vi "4.2.vi"() -> ()   [LabVIEW 2016]
panel:
  out "波形图":dbl[][](graph)
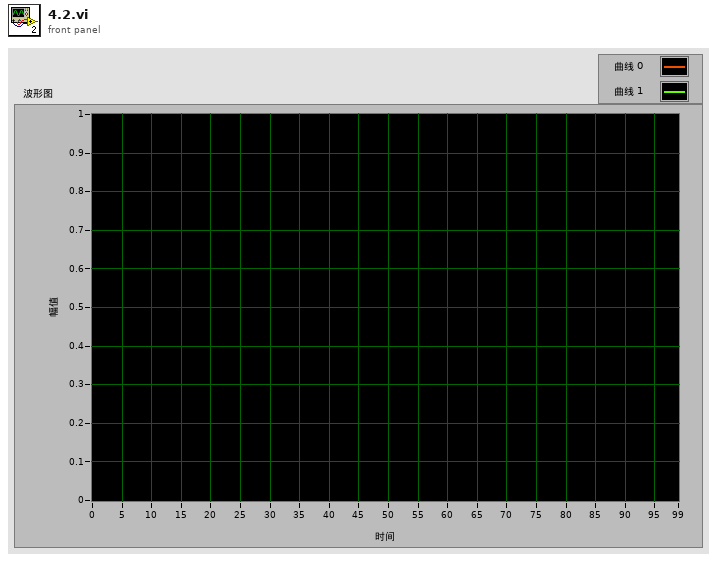
[diagram p1: front panel]
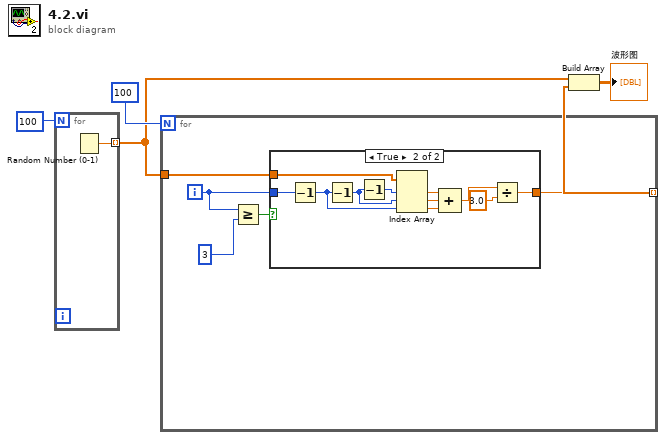
[diagram p0: block diagram]
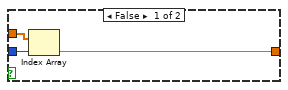
[diagram p2: hidden frame]
diagram:
  n1 = for {
    N: 100 -> [_]
    tunnel: [w6] -> w2 mode=indexing
    n2 = Random Number (0-1)() -> (number: 0 to 1=w6:dbl)
  }
  n3 = for {
    N: 100 -> [_]
    tunnel: [w7] -> w1 mode=indexing
    tunnel: w2 -> [w8]
    i -> [w9]
    n4 = Greater Or Equal?(x=w9, y=3) -> (x >= y?=w11:bool)
    n5 = case shown="True" w11 {
      tunnel: w9 -> [w13 w17]
      tunnel: w8 -> [w14 w16]
      tunnel: [w12 w15] -> w7
      frame False {
        n6 = Index Array(array=w14, index=w13) -> (element=w12:dbl)
      }
      frame True {
        n7 = Decrement(x=w17) -> (x-1=w19:i32)
        n8 = Decrement(x=w19) -> (x-1=w21:i32)
        n9 = Decrement(x=w21) -> (x-1=w20:i32)
        n10 = Index Array(array=w16, index #1=w20, index #2=w21, index #3=w19) -> (element #1=w22:dbl, element #2=w23:dbl, element #3=w24:dbl)
        n11 = Compound Arithmetic op=ADD(w22, w23, w24) -> (w25:dbl)
        n12 = Divide(x=w25, y=3.0) -> (x/y=w15:dbl)
      }
    }
  }
  n13 = Build Array(w2, w1) -> (→"波形图":dbl[][])
